vi "Terminate Condition A.vi"(6 "Burner ON":bool, 8 "error in":errorcluster, 11 "PLC Data In":T1 {"PLC Data - LDO"."Timing"."Absolute Time" format="%<%H:%M:%S%3u>t"; "PLC Data - LDO"."Timing"."Display Time" format="%#.20f"; "PLC Data - LDO"."Timing"."Test Time Ref" format="%#.20f"; "PLC Data - LDO"."Timing"."Precondition Time Ref" format="%#.20f"; "PLC Data - LDO"."Timing"."First Call Time Ref" format="%#.20f"; "PLC Data - FVIR"."Timing"."Absolute Time" format="%<%H:%M:%S%3u>t"; "PLC Data - FVIR"."Timing"."Display Time" format="%#.20f"; "PLC Data - FVIR"."Timing"."Test Time Ref" format="%#.20f"; "PLC Data - FVIR"."Timing"."Precondition Time Ref" format="%#.20f"; "PLC Data - FVIR"."Timing"."First Call Time Ref" format="%#.20f"}) -> (0 "error out":errorcluster, 3 "PLC Data Out":T1 {"PLC Data - LDO"."Timing"."Absolute Time" format="%<%H:%M:%S%3u>t"; "PLC Data - LDO"."Timing"."Display Time" format="%#.20f"; "PLC Data - LDO"."Timing"."Test Time Ref" format="%#.20f"; "PLC Data - LDO"."Timing"."Precondition Time Ref" format="%#.20f"; "PLC Data - LDO"."Timing"."First Call Time Ref" format="%#.20f"; "PLC Data - FVIR"."Timing"."Absolute Time" format="%<%H:%M:%S%3u>t"; "PLC Data - FVIR"."Timing"."Display Time" format="%#.20f"; "PLC Data - FVIR"."Timing"."Test Time Ref" format="%#.20f"; "PLC Data - FVIR"."Timing"."Precondition Time Ref" format="%#.20f"; "PLC Data - FVIR"."Timing"."First Call Time Ref" format="%#.20f"})   [LabVIEW 2023]
uses:
  Modbus/Modbus PLC Data All.ctl
  Modbus/Modbus FVIR Control.ctl
  Modbus/Modbus Timing.ctl
  <vilib>/Utility/miscctls.llb/LVDateTimeRec.ctl
  Modbus/Modbus LDO Control.ctl
  WritingDataFile/Data to Save.ctl
  Terminate Conditions Cluster.ctl
  Terminate Condition ENUM.ctl
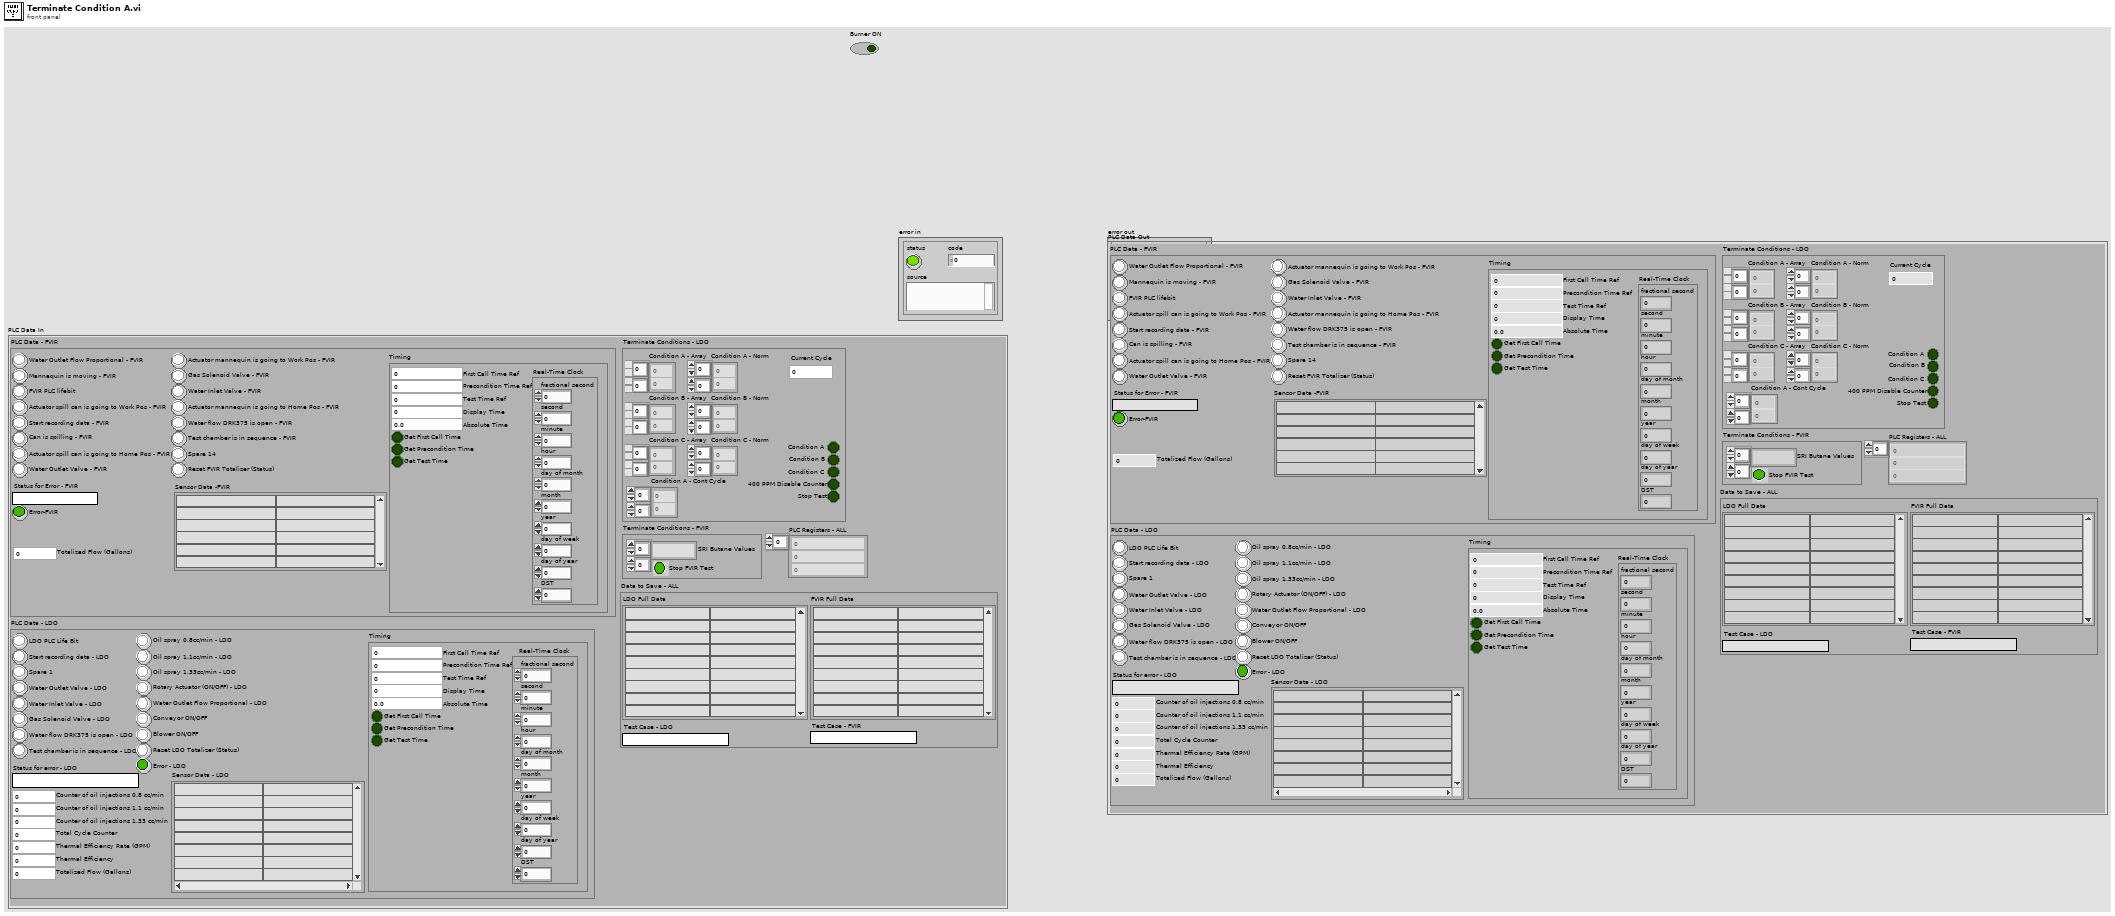
[diagram p1: front panel]
types:
  T1 = typedef "Modbus PLC Data All.ctl" = cluster{"PLC Data - FVIR":T2, "PLC Data - LDO":T5, "PLC Registers - ALL":i16[], "Data to Save - ALL":T6, "Terminate Conditions - LDO":T7, "Terminate Conditions - FVIR":cluster{"SRI Butane Values":string[][], "Stop FVIR Test":bool}}
  T2 = typedef "Modbus FVIR Control.ctl" = cluster{"Reset FVIR Totalizer (Status)":bool, "Spare 14":bool, "Actuator mannequin is going to Work Pos - FVIR":bool, "Actuator mannequin is going to Home Pos - FVIR":bool, "Test chamber is in sequence - FVIR ":bool, "Water flow DRK375 is open - FVIR":bool, "Gas Solenoid Valve - FVIR":bool, "Water Inlet Valve - FVIR":bool, "Water Outlet Flow Proportional - FVIR":bool, "Start recording data - FVIR":bool, "Actuator spill can is going to Work Pos - FVIR":bool, "Actuator spill can is going to Home Pos - FVIR":bool, "Water Outlet Valve - FVIR":bool, "Can is spilling - FVIR":bool, "Mannequin is moving - FVIR":bool, "FVIR PLC lifebit":bool, "Status for Error - FVIR":string, "Error-FVIR":bool, "Sensor Data -FVIR":string[][], "Totalized Flow (Gallons)":dbl, "Timing":T3}
  T3 = typedef "Modbus Timing.ctl" = cluster{"First Call Time Ref":dbl, "Precondition Time Ref":dbl, "Test Time Ref":dbl, "Get First Call Time":bool, "Get Precondition Time":bool, "Get Test Time":bool, "Display Time":dbl, "Real-Time Clock":T4, "Absolute Time":dbl}
  T4 = typedef "LVDateTimeRec.ctl" = cluster{"fractional second":dbl, "second":i32, "minute":i32, "hour":i32, "day of month":i32, "month":i32, "year":i32, "day of week":i32, "day of year":i32, "DST":i32}
  T5 = typedef "Modbus LDO Control.ctl" = cluster{"LDO PLC Life Bit":bool, "Start recording data - LDO":bool, "Spare 1":bool, "Water Outlet Valve - LDO":bool, "Water Inlet Valve - LDO":bool, "Gas Solenoid Valve - LDO":bool, "Water flow DRK375 is open - LDO":bool, "Test chamber is in sequence - LDO":bool, "Oil spray 0.8cc/min - LDO":bool, "Oil spray 1.1cc/min - LDO":bool, "Oil spray 1.33cc/min - LDO":bool, "Rotary Actuator (ON/OFF) - LDO":bool, "Water Outlet Flow Proportional - LDO":bool, "Conveyor ON/OFF":bool, "Blower ON/OFF":bool, "Reset LDO Totalizer (Status)":bool, "Status for error - LDO":string, "Error - LDO":bool, "Sensor Data - LDO":string[][], "Thermal Efficiency Rate (GPM)":dbl, "Thermal Efficiency":dbl, "Totalized Flow (Gallons)":dbl, "Counter of oil injections 1.33 cc/min":u16, "Total Cycle Counter":u16, "Counter of oil injections 1.1 cc/min":u16, "Counter of oil injections 0.8 cc/min":u16, "Timing":T3}
  T6 = typedef "Data to Save.ctl" = cluster{"LDO Full Data":string[][], "FVIR Full Data":string[][], "Test Case - FVIR":string, "Test Case - LDO":string}
  T7 = typedef "Terminate Conditions Cluster.ctl" = cluster{"Condition B - Array":dbl[][], "Current Cycle":u16, "Condition C - Array":dbl[][], "Condition A - Array":dbl[][], "400 PPM Disable Counter":bool, "Condition A - Norm":dbl[][], "Condition B - Norm":dbl[][], "Condition C - Norm":dbl[][], "Condition A":bool, "Condition B":bool, "Condition C":bool, "Condition A - Cont Cycle":dbl[][], "Stop Test":bool}
  T8 = typedef "Terminate Condition ENUM.ctl" = enum16{"Condition A", "Condition B", "Condition C"}
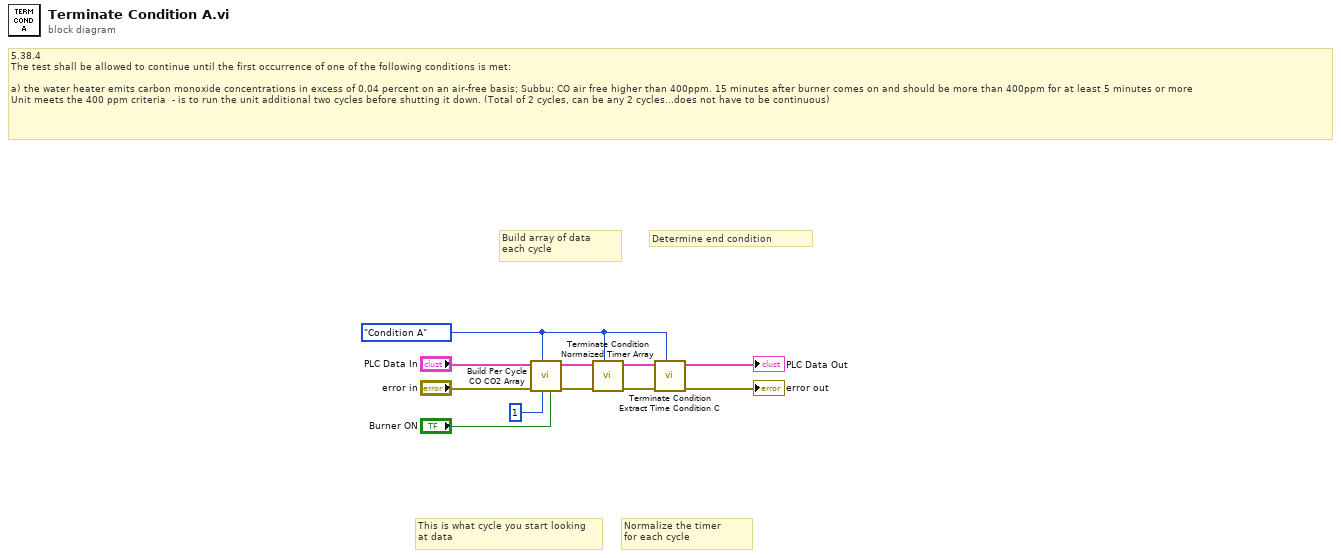
[diagram p0: block diagram]
diagram:
  w4 = Terminate_Condition_ENUM."Condition A" ("Conditions")
  # "Determine end condition"
  # "Normalize the timer\nfor each cycle"
  # "Build array of data\neach cycle"
  # "This is what cycle you start looking\nat data"
  # "5.38.4\nThe test shall be allowed to continue until the first occurrence of one of the following conditions is met: \n\na) the water heater emits carbon monoxide concentrations in excess of 0.04 percent on an air-free basis; Subbu: CO air free higher than 400ppm. 15 minutes after burner comes on and should be more than 400ppm for at least 5 minutes or more\nUnit meets the 400 ppm criteria  - is to run the unit additional two cycles before shutting it down. (Total of 2 cycles, can be any 2 cycles...does not have to be continuous)"
  n1 = call "Build Per Cycle CO CO2 Array.vi"("Burner ON"="Burner ON", "Start Analyzing Cycles at"=u16 1, "Conditions"=w4, "error in"="error in", "PLC Data In"="PLC Data In") -> ("error out"=w8:errorcluster, "PLC Data Out"=w5:T1)  [unwired: 5 in]
  n2 = call "Terminate Condition Normaized Timer Array.vi"("Conditions"=w4, "error in"=w8, "PLC Data In"=w5) -> ("error out"=w6:errorcluster, "PLC Data Out"=w7:T1)  [unwired: 7 in]
  n3 = call "Terminate Condition Extract Time Condition C.vi"("Conditions"=w4, "error in"=w6, "PLC Data In"=w7) -> ("error out"=→"error out":errorcluster, "PLC Data Out"=→"PLC Data Out":T1)  [unwired: 7 in]
